vi "Array-Circular Subarray.vi"(8 "Npts":i32, 9 "Offset (in)":i32, 11 "Array":dbl[](array[numeric])) -> (1 "Offset (out)":i32, 2 "Subarray":dbl[](array[numeric]))   [LabVIEW 2020]
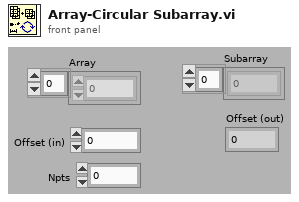
[diagram p1: front panel]
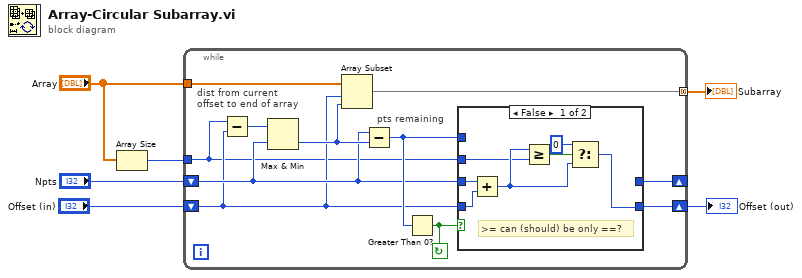
[diagram p0: block diagram]
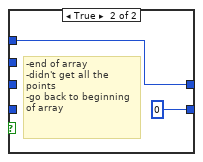
[diagram p2: hidden frame]
diagram:
  n1 = Array Size(array="Array") -> (size(s)=w3:i32)
  n2 = while {
    tunnel: "Array" -> [w17]
    tunnel: [w9] -> w5 mode=concatenating
    tunnel: w3 -> [w7]
    shift-right: [w8] -> w1
    shift-left: "Offset (in)" -> [w12]
    shift-right: [w10] -> _
    shift-left: "Npts" -> [w13]
    stop <- w11 continue-if-true
    # "pts remaining"
    # "dist from current offset to end of array"
    n3 = Subtract(x=w7, y=w12) -> (x-y=w15:i32)
    n4 = Max & Min(x=w15, y=w13) -> (min(x,y)=w16:i32)  [unwired: 1 out]
    n5 = Array Subset(array=w17, index=w12, length=w16) -> (w9:dbl[])
    n6 = Subtract(x=w13, y=w16) -> (x-y=w14:i32)
    n7 = Greater Than 0?(x=w14) -> (x > 0?=w11:bool)
    n8 = case shown="False" w11 {
      tunnel: w14 -> [_ w26]
      tunnel: w13 -> [w24 _]
      tunnel: w12 -> [w23 _]
      tunnel: [_ w26] -> w10
      tunnel: [w19 0] -> w8
      tunnel: w7 -> [w18 _]
      frame False {
        # ">= can (should) be only ==?"
        n9 = Add(x=w24, y=w23) -> (x+y=w20:i32)
        n10 = Greater Or Equal?(x=w20, y=w18) -> (x >= y?=w22:bool)
        n11 = Select(t=0, s=w22, f=w20) -> (s? t:f=w19:i32)
      }
      frame True {
        # "-end of array\n-didn't get all the points\n-go back to beginning of array"
      }
    }
  }
  "Offset (out)" <- w1
  "Subarray" <- w5
